vi "excitation controls.vi"() -> ()   [LabVIEW 2015]
panel:
  out "Measured Power (mW)":T1
  in  "Power (mW)":T1
  in  "Excitation":T2
  in  "Radio Buttons":T3(radio)
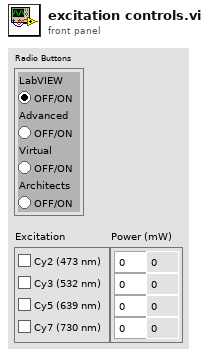
[diagram p1: front panel]
types:
  T1 = cluster{"Cy2":dbl, "Cy3":dbl, "Cy5":dbl, "Cy7":dbl}
  T2 = cluster{"Cy2 (473 nm)":bool, "Cy3 (532 nm)":bool, "Cy5 (639 nm)":bool, "Cy7 (730 nm)":bool}
  T3 = enum32{"Radio Selection 1", "Radio Selection 2", "Radio Selection 3", "Radio Selection 4"}
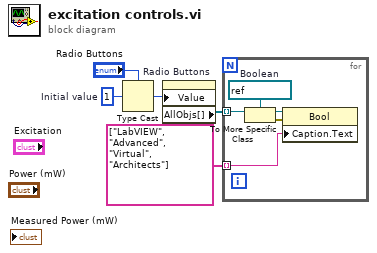
[diagram p0: block diagram]
diagram:
  w1 = 1  # Initial value
  n1 = Type Cast(type="Radio Buttons", x=w1) -> (*(type *) &x=w2:T3)
  n2 = property on="Radio Buttons" class="RadioBtnsControl (strict)"("Value"=w2) -> ("AllObjs[]"=w4:refnum<vi>[])  [unwired: 2 in, 2 out]
  n3 = for {
    tunnel: w4 -> [w10] mode=indexing
    tunnel: string[] ["LabVIEW", "Advanced", "Virtual", "Architects"] -> [w6] mode=indexing
    w8 = refnum<vi> refnum  # Boolean
    n4 = To More Specific Class(target class=w8, reference=w10) -> (specific class reference=w9:refnum<vi>, error out=w7:errorcluster)  [unwired: 1 in]
    n5 = property class="Bool"(reference=w9, error in=w7, "Caption.Text"=w6) -> ()  [unwired: 2 out]
  }
